vi "Actor Core.vi"(8 "error in (no error)":errorcluster, 11 "Actor in":refnum<class "Actor1_GUI_N_4.0.0.lvclass">) -> (0 "error out":errorcluster, 3 "Actor out":refnum<class "Actor.lvclass">)   [LabVIEW 2014, in "Actor1_GUI_N_4.0.0.lvlib" / "Actor1_GUI_N_4.0.0.lvclass"]
uses:
  <resource>/Framework/Providers/Open_GDS/ClassProviders/ActorFramework/4.0.0/Actor1_GUI_N_4.0.0/Actor1_GUI_N_4.0.0_class/Actor1_GUI_N_4.0.0.lvclass
  <vilib>/ActorFramework/Actor/Actor.lvclass
  <resource>/Framework/Providers/Open_GDS/ClassProviders/ActorFramework/4.0.0/Actor1_GUI_N_4.0.0/Actor1_GUI_N_4.0.0_class/Actor1_GUI_N_4.0.0.lvclass/Actor1_GUI_N_4.0.0.ctl
panel:
  out "Waveform Graph":dynamicdata(graph)
  in  "Freq":dbl(slide)=10.1 scale=0.0..20.0
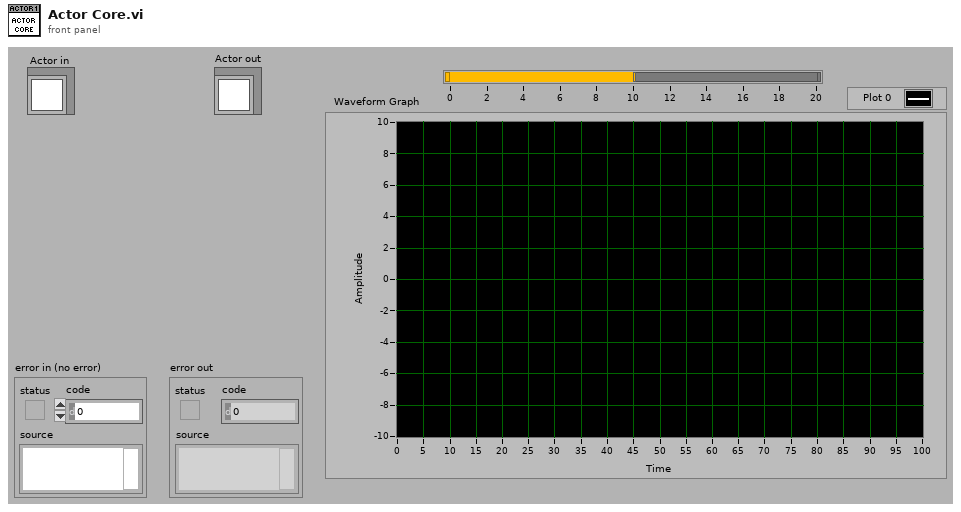
[diagram p1: front panel]
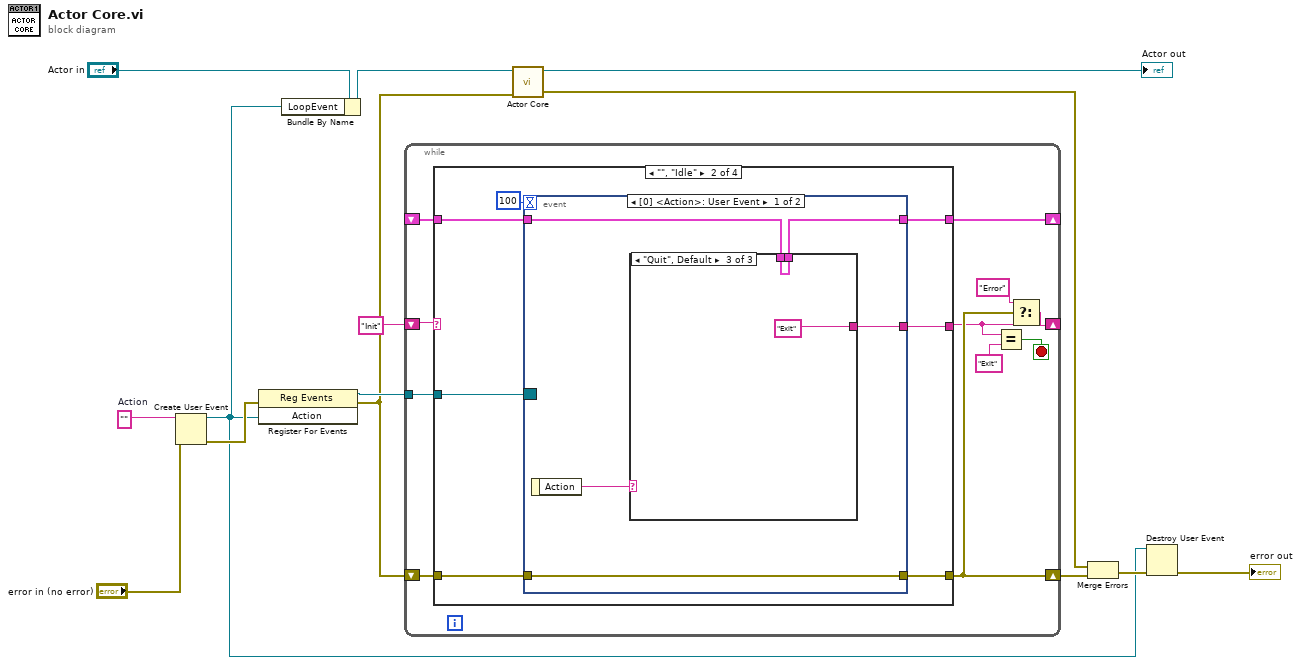
[diagram p0: block diagram]
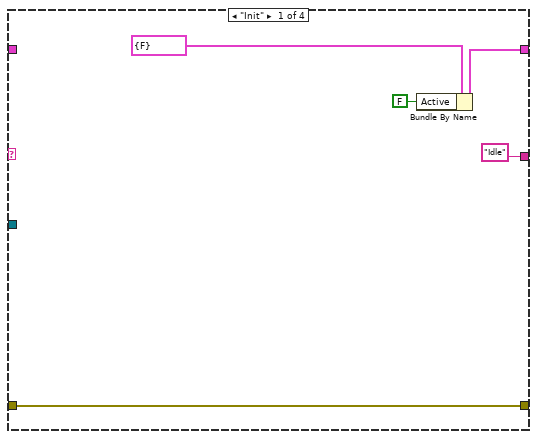
[diagram p2: hidden frame]
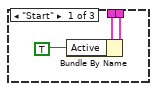
[diagram p3: hidden frame]
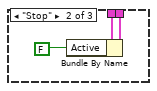
[diagram p4: hidden frame]
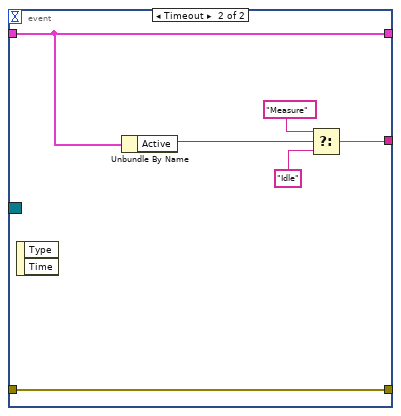
[diagram p5: hidden frame]
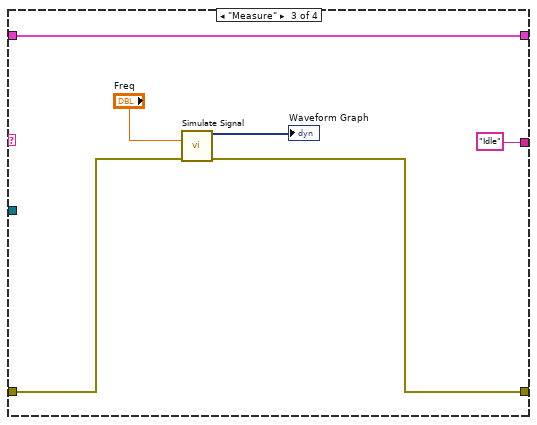
[diagram p6: hidden frame]
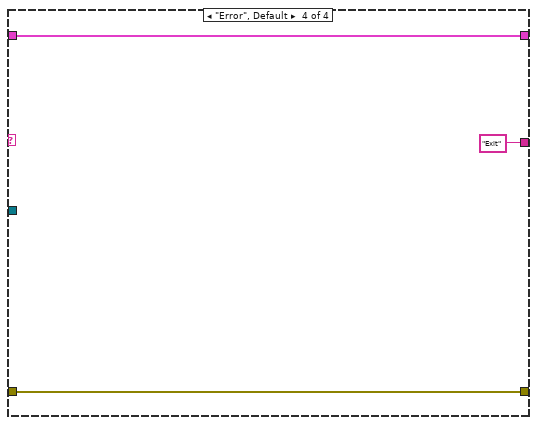
[diagram p7: hidden frame]
diagram:
  w5 = ""  # Action
  n1 = Create User Event(user event datatype=w5, error in="error in (no error)") -> (user event=w1:refnum<user-event>, error out=w9:errorcluster)
  n2 = register-events(error in=w9, w1) -> (reference out=w10:refnum<event-registration>, error out=w8:errorcluster)  [unwired: 1 in]
  n3 = Bundle By Name(cluster="Actor in", "LoopEvent"=w1) -> (w12:refnum<class "Actor1_GUI_N_4.0.0.lvclass">)
  n4 = while {
    tunnel: w10 -> [w25]
    shift-right: [w20] -> _
    shift-left: "Init" -> [w24]
    shift-right: [w21] -> w7
    shift-left: w8 -> [w23]
    shift-right: [w17] -> _
    shift-left: _ -> [w16]
    stop <- w22 stop-if-true
    n5 = case shown="\"\", \"Idle\"" w24 {
      tunnel: w25 -> [_ w37 _ _]
      tunnel: ["Idle" w36 "Idle" "Exit" ("y")] -> w18
      tunnel: w23 -> [w29 w33 w57 w64]
      tunnel: [w29 w32 w58 w64] -> w21
      tunnel: [w26 w34 w60 w63] -> w17
      tunnel: w16 -> [_ w31 w60 w63]
      frame "Init" {
        n6 = Bundle By Name(cluster=cluster{"Active":bool} {"Active"=FALSE}, "Active"=FALSE) -> (w26:cluster{"Active":bool})
      }
      frame "", "Idle" {
        n7 = event shown="[0] <Action>: User Event" {
          selector: w37 -> [_ _]
          dyn-events: _ -> [_ _]
          timeout: 100 -> [_ _]
          tunnel: [w41 w51] -> w36
          tunnel: w31 -> [w40 w55]
          tunnel: [w39 w55] -> w34
          tunnel: w33 -> [w38 w56]
          tunnel: [w38 w56] -> w32
          event User Event {
            n8 = event-data() -> ("Action"=w42:string)  [unwired: 1 in]
            n9 = case shown="\"Quit\", Default" w42 {
              tunnel: [_ _ "Exit" ("y")] -> w41
              tunnel: w40 -> [w45 w48 w49]
              tunnel: [w44 w47 w49] -> w39
              frame "Start" {
                n10 = Bundle By Name(cluster=w45, "Active"=TRUE) -> (w44:cluster{"Active":bool})
              }
              frame "Stop" {
                n11 = Bundle By Name(cluster=w48, "Active"=FALSE) -> (w47:cluster{"Active":bool})
              }
              frame "Quit", Default {
              }
            }
          }
          event Timeout {
            n12 = event-data() -> ()  [unwired: 1 in, 2 out]
            n13 = Unbundle By Name(w55) -> ("Active"=w54:bool)
            n14 = Select(t="Measure", s=w54, f="Idle") -> (s? t:f=w51:string)
          }
        }
      }
      frame "Measure" {
        n15 = call "Simulate Signal"("Frequency"="Freq", "error in (no error)"=w57) -> ("Sine with Uniform Noise"=→"Waveform Graph":dynamicdata, "error out"=w58:errorcluster)  [unwired: 12 in]
      }
      frame "Error", Default {
      }
    }
    n16 = Equal?(x=w18, y="Exit") -> (x = y?=w22:bool)
    n17 = Select(t="Error", s=w21, f=w18) -> (s? t:f=w20:string)
  }
  n18 = call-parent "Actor Core.vi"("error in"=w8, "Actor in"=w12) -> ("error out"=w6:errorcluster, "Actor out"=→"Actor out":refnum<class "Actor.lvclass">)  [unwired: 8 in]
  n19 = Merge Errors(w6, w7) -> (w3:errorcluster)
  n20 = Destroy User Event(user event=w1, error in=w3) -> (error out=→"error out":errorcluster)
